vi "PROXY_save_database_password.vi"(7 "error_in":errorcluster, 9 "new_password":string, 10 "all_config_info_in":T1) -> (0 "error_out":errorcluster, 3 "all_config_info_out":T1)   [LabVIEW 2020]
uses:
  typedef/PROXY_all_config_info.ctl
  typedef/PROXY_main_ini_file.ctl
  queues/typedef/PROXY_queue_refnums.ctl
  queues/typedef/STATION_queue_element.ctl
  STATION/ST_SQL_sequence_state.ctl
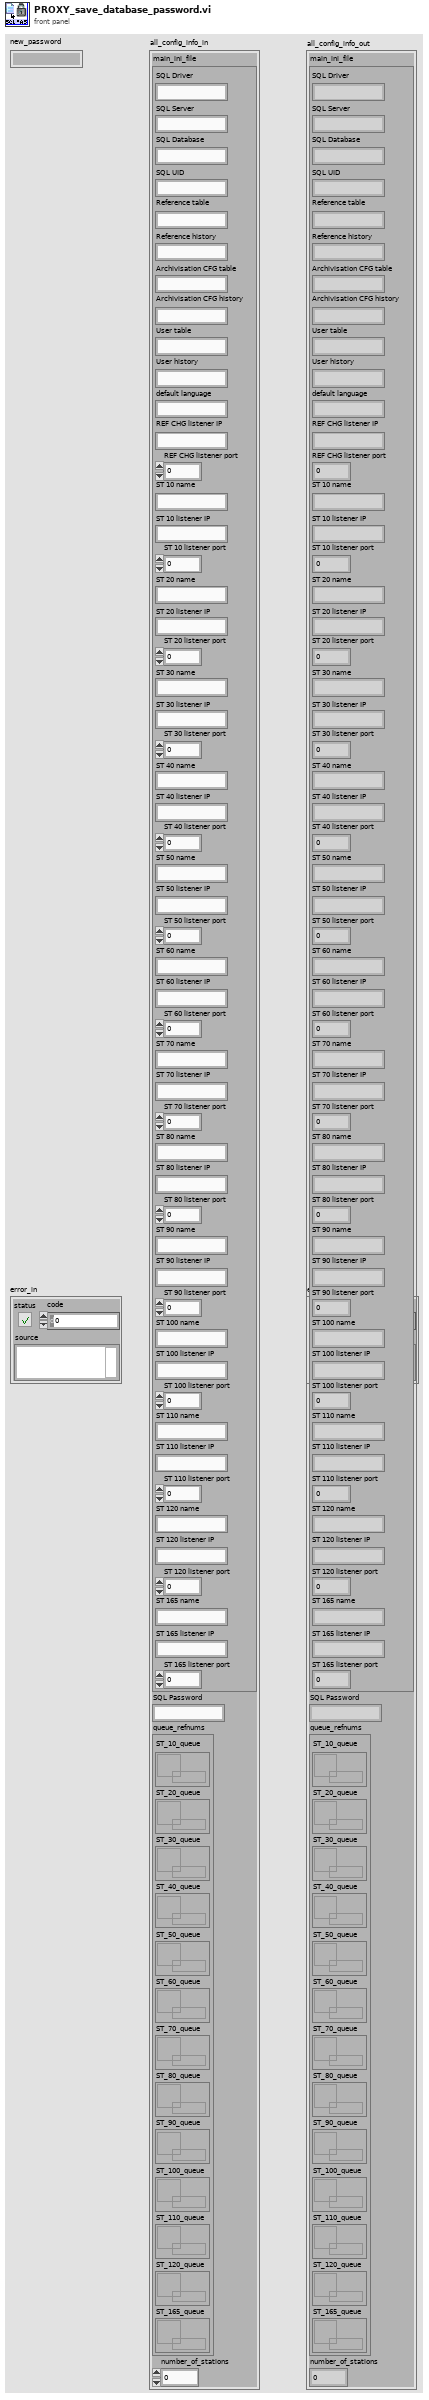
[diagram p1: front panel]
types:
  T1 = typedef "PROXY_all_config_info.ctl" = cluster{"main_ini_file":T2, "SQL Password":string, "queue_refnums":T3, "number_of_stations":i32}
  T2 = typedef "PROXY_main_ini_file.ctl" = cluster{"SQL Driver":string, "SQL Server":string, "SQL Database":string, "SQL UID":string, "Reference table":string, "Reference history":string, "Archivisation CFG table":string, "Archivisation CFG history":string, "User table":string, "User history":string, "default language":string, "REF CHG listener IP":string, "REF CHG listener port":u16, "ST 10 name":string, "ST 10 listener IP":string, "ST 10 listener port":u16, "ST 20 name":string, "ST 20 listener IP":string, "ST 20 listener port":u16, "ST 30 name":string, "ST 30 listener IP":string, "ST 30 listener port":u16, "ST 40 name":string, "ST 40 listener IP":string, "ST 40 listener port":u16, "ST 50 name":string, "ST 50 listener IP":string, "ST 50 listener port":u16, "ST 60 name":string, "ST 60 listener IP":string, "ST 60 listener port":u16, "ST 70 name":string, "ST 70 listener IP":string, "ST 70 listener port":u16, "ST 80 name":string, "ST 80 listener IP":string, "ST 80 listener port":u16, "ST 90 name":string, "ST 90 listener IP":string, "ST 90 listener port":u16, "ST 100 name":string, "ST 100 listener IP":string, "ST 100 listener port":u16, "ST 110 name":string, "ST 110 listener IP":string, "ST 110 listener port":u16, "ST 120 name":string, "ST 120 listener IP":string, "ST 120 listener port":u16, "ST 165 name":string, "ST 165 listener IP":string, "ST 165 listener port":u16}
  T3 = typedef "PROXY_queue_refnums.ctl" = cluster{"ST_10_queue":refnum<queue>, "ST_20_queue":refnum<queue>, "ST_30_queue":refnum<queue>, "ST_40_queue":refnum<queue>, "ST_50_queue":refnum<queue>, "ST_60_queue":refnum<queue>, "ST_70_queue":refnum<queue>, "ST_80_queue":refnum<queue>, "ST_90_queue":refnum<queue>, "ST_100_queue":refnum<queue>, "ST_110_queue":refnum<queue>, "ST_120_queue":refnum<queue>, "ST_165_queue":refnum<queue>}
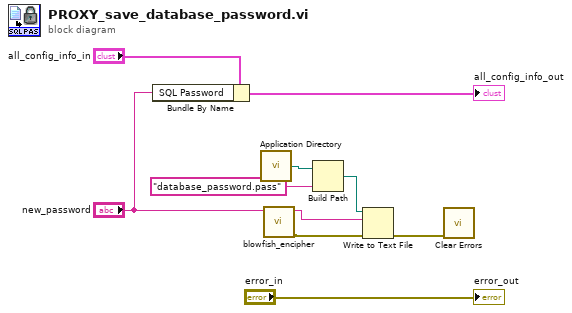
[diagram p0: block diagram]
diagram:
  n1 = Bundle By Name(cluster="all_config_info_in", "SQL Password"="new_password") -> (→"all_config_info_out":T1)
  n2 = call <vilib>:"Application Directory.vi"() -> ("Application Directory"=w9:path)
  n3 = call "blowfish_encipher.vi"("Input Text"="new_password") -> ("error out"=w5:errorcluster, "Output Text"=w4:string)  [unwired: 9 in]
  n4 = Build Path(base path=w9, name or relative path="database_password.pass") -> (appended path=w7:path)
  n5 = Write to Text File(file (use dialog)=w7, text=w4, error in=w5) -> (error out=w6:errorcluster)  [unwired: 1 in, 2 out]
  n6 = call <vilib>:"Clear Errors.vi"("error in (no error)"=w6) -> ()  [unwired: 5 in, 2 out]
  "error_out" <- "error_in"
